vi "Force Include Target Types.vi"(10 "Target Types to include":string[](array[string]), 11 "Original Target Types":string[](array[string])) -> (3 "Final Target Types":string[](array[string]))   [LabVIEW 2020]
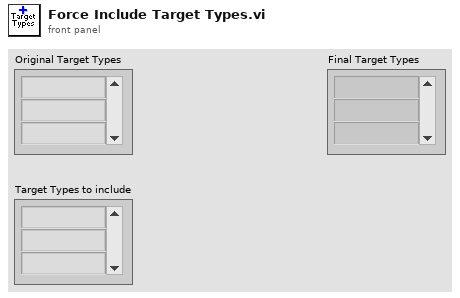
[diagram p1: front panel]
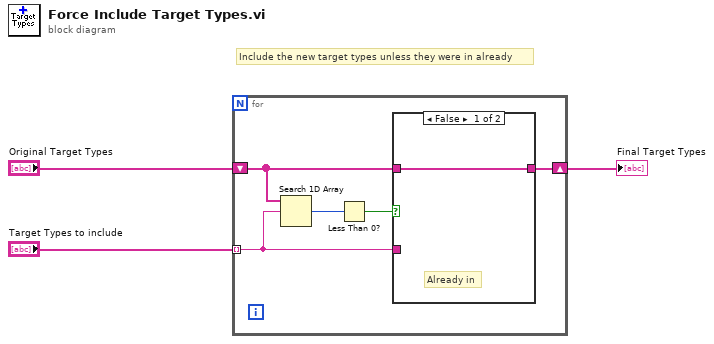
[diagram p0: block diagram]
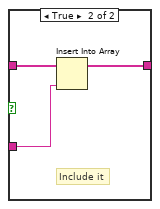
[diagram p2: hidden frame]
diagram:
  # "Include the new target types unless they were in already"
  n1 = for {
    shift-right: [w6] -> w1
    shift-left: "Original Target Types" -> [w5]
    tunnel: "Target Types to include" -> [w4] mode=indexing
    n2 = Search 1D Array(1D array=w5, element=w4) -> (index of element=w8:i32)  [unwired: 1 in]
    n3 = Less Than 0?(x=w8) -> (x < 0?=w7:bool)
    n4 = case shown="False" w7 {
      tunnel: [w9 w11] -> w6
      tunnel: w5 -> [w9 w12]
      tunnel: w4 -> [_ w10]
      frame False {
        # "Already in"
      }
      frame True {
        # "Include it"
        n5 = Insert Into Array "Insert Into Array"(array=w12, new element=w10) -> (w11:string[])  [unwired: 1 in]
      }
    }
  }
  "Final Target Types" <- w1
